vi "MyFunction.vi"(9 "c":dbl, 10 "b":dbl, 11 "a":dbl) -> (2 "x*y":dbl)   [LabVIEW 2020]
doc: "hjsgafkjsflkjahkjashdkjascnvccjhgjhdgj"
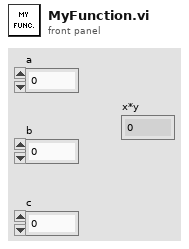
[diagram p1: front panel]
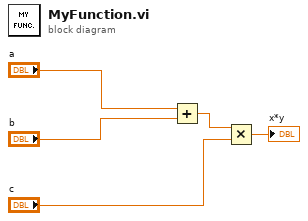
[diagram p0: block diagram]
diagram:
  n1 = Add(x="a", y="b") -> (x+y=w3:dbl)
  n2 = Multiply(x=w3, y="c") -> (x*y=→"x*y":dbl)
